vi "Set Limits on Configure Device.vi"(8 "error in (no error)":errorcluster, 10 "cluster":T1, 11 "Toggle 6 in":refnum<class "Toggle 6.lvclass">) -> (0 "error out":errorcluster, 3 "Toggle 6 out":refnum<class "Toggle 6.lvclass">)   [LabVIEW 2020, in "Toggle 6.lvclass"]
uses:
  Toggle 6.lvclass
  C:/Sandbox/Git_Sandbox/WiSpry Test Framework source code (LV20)/WiSpry Test Framework/Devices/Device.lvclass
  Controls/Configure decive refs cluster.ctl
  Controls/EFuse modes enum.ctl
  Controls/Set limt states.ctl
  <vilib>/Utility/miscctls.llb/LVMinMaxIncTypeDef.ctl
  <vilib>/Utility/miscctls.llb/LVOutOfRangeActionTypeDef.ctl
  Instruments/Power Supply/Power Supply.lvclass
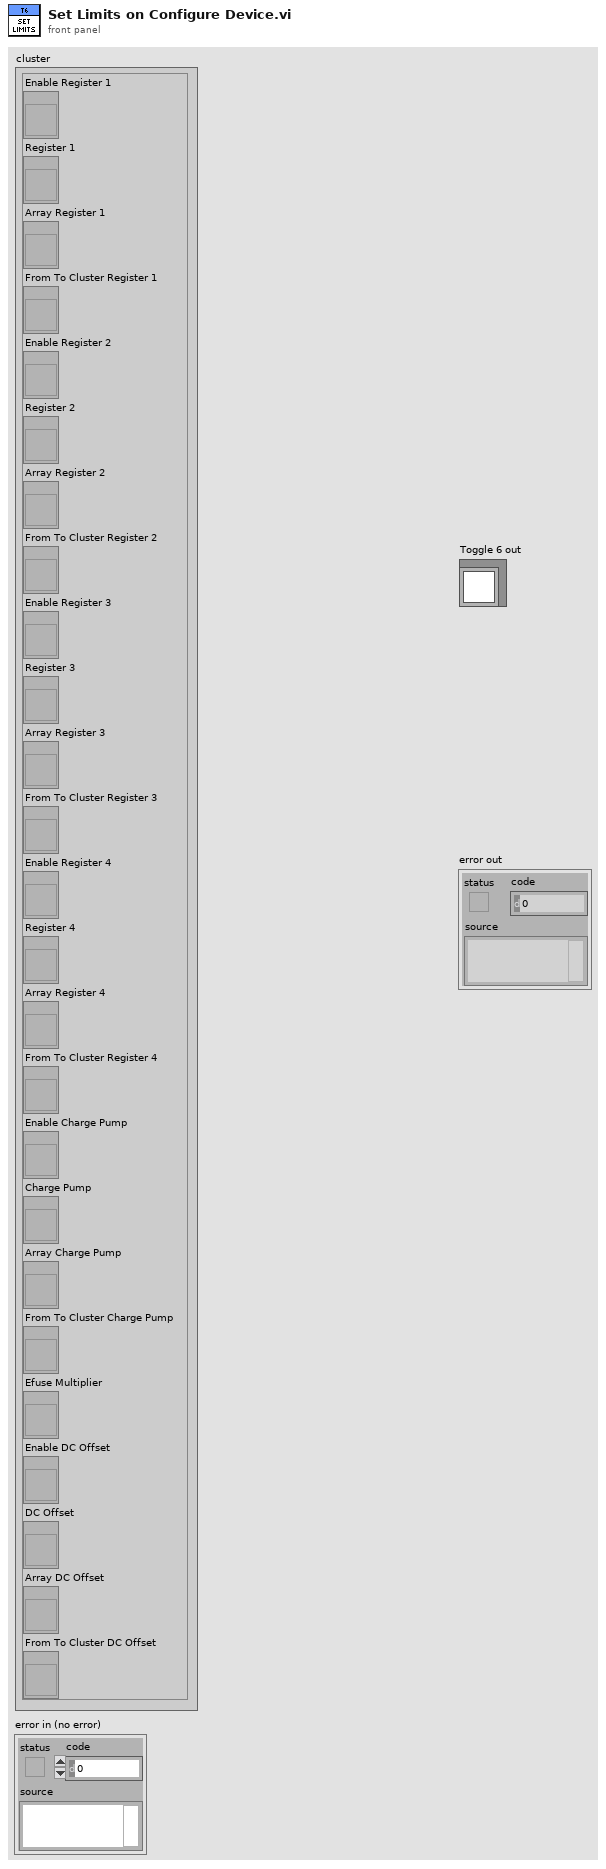
[diagram p1: front panel]
types:
  T1 = typedef "Toggle 6.lvclass/Configure decive refs cluster.ctl" = cluster{"Enable Register 1":refnum<vi>, "Register 1":refnum<vi>, "Array Register 1":refnum<vi>, "From To Cluster Register 1":refnum<vi>, "Enable Register 2":refnum<vi>, "Register 2":refnum<vi>, "Array Register 2":refnum<vi>, "From To Cluster Register 2":refnum<vi>, "Enable Register 3":refnum<vi>, "Register 3":refnum<vi>, "Array Register 3":refnum<vi>, "From To Cluster Register 3":refnum<vi>, "Enable Register 4":refnum<vi>, "Register 4":refnum<vi>, "Array Register 4":refnum<vi>, "From To Cluster Register 4":refnum<vi>, "Enable Charge Pump":refnum<vi>, "Charge Pump":refnum<vi>, "Array Charge Pump":refnum<vi>, "From To Cluster Charge Pump":refnum<vi>, "Efuse Multiplier":refnum<vi>, "Enable DC Offset":refnum<vi>, "DC Offset":refnum<vi>, "Array DC Offset":refnum<vi>, "From To Cluster DC Offset":refnum<vi>}
  T2 = typedef "Toggle 6.lvclass/Capacitor register.ctl" = cluster{"Register":u32, "Beam":dbl, "Trimmer":dbl}
  T3 = typedef "Toggle 6.lvclass/Set limt states.ctl" = enum16{"Reg 1", "Reg 2", "Reg 3", "Reg 4", "CP", "Efuse", "DC Offset", "Info", "Done"}
  T4 = typedef "LVOutOfRangeActionTypeDef.ctl" = cluster{"Out of Range Action Minimum":u8, "Out of Range Action Maximum":u8, "Out of Range Action Increment":u8}
  T5 = typedef "LVMinMaxIncTypeDef.ctl" = cluster{"Minimum":dbl, "Maximum":dbl, "Increment":dbl}
  T6 = enum8{"Enabled", "Disabled", "Disabled and Grayed Out"}
  T7 = typedef "Toggle 6.lvclass/Parameter Cluster.ctl" = cluster{"Enable":bool, "Register Number":u32, "Use Array":bool, "Array":dbl[], "To From Cluster":cluster{"From":dbl, "To":dbl, "Step":dbl}}
  T8 = typedef "Toggle 6.lvclass/Charge Pump Information cluster.ctl" = cluster{"Min":dbl, "Max":dbl, "Step":dbl, "Default":dbl}
  T9 = typedef "Toggle 6.lvclass/EFuse modes enum.ctl" = enum16{"On", "Off", "Both On and Off"}
  T10 = typedef "Device.lvclass/DC Offset Cluster.ctl" = cluster{"Enable":bool, "Use Array":bool, "Array":dbl[], "To From Cluster":cluster{"From":dbl, "To":dbl, "Step":dbl}, "Current Value":dbl, "DC Offset":refnum<class "Power Supply.lvclass">}
  T11 = typedef "Device.lvclass/Device Information Cluster.ctl" = cluster{"Device Info":string[][], "Default Values":T12[], "Fetched info":string[][]}
  T12 = typedef "PIC-Device.lvclass/Register to Write.ctl" = cluster{"Register":u32, "Value":u32, "Dev Address":u32, "Physical Adress":u32}
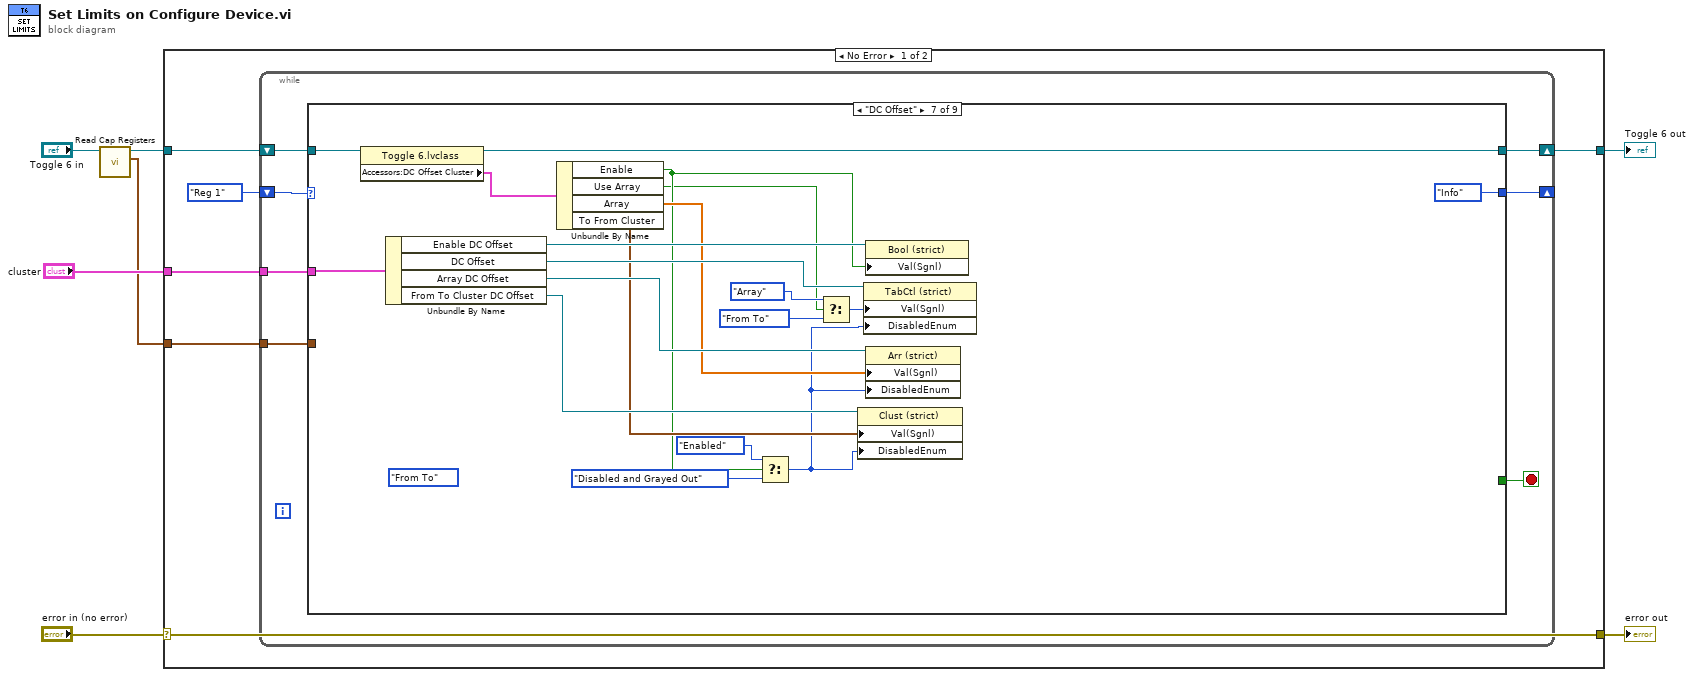
[diagram p0: block diagram]
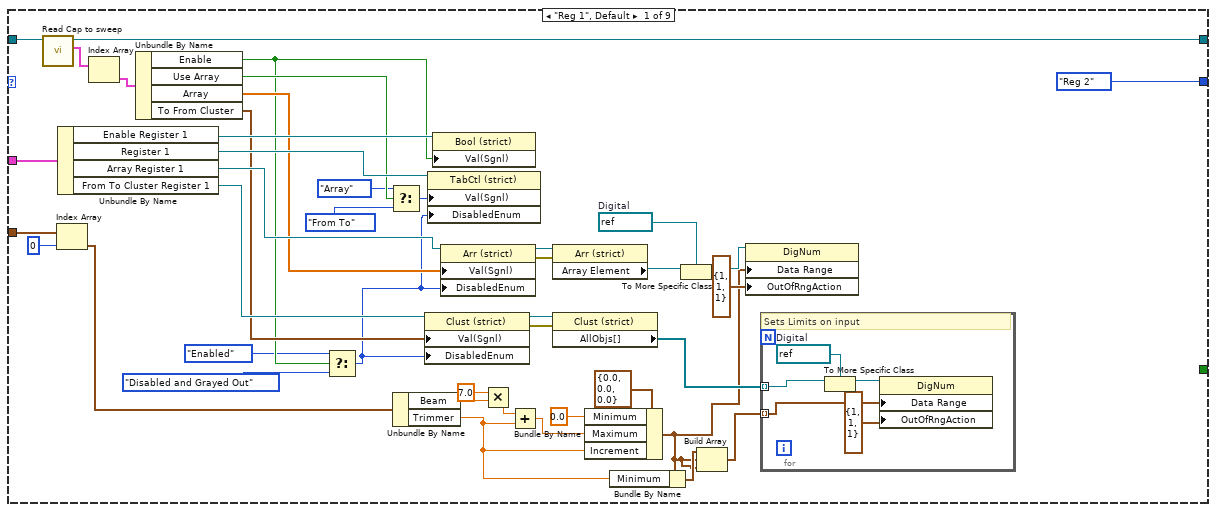
[diagram p2: hidden frame]
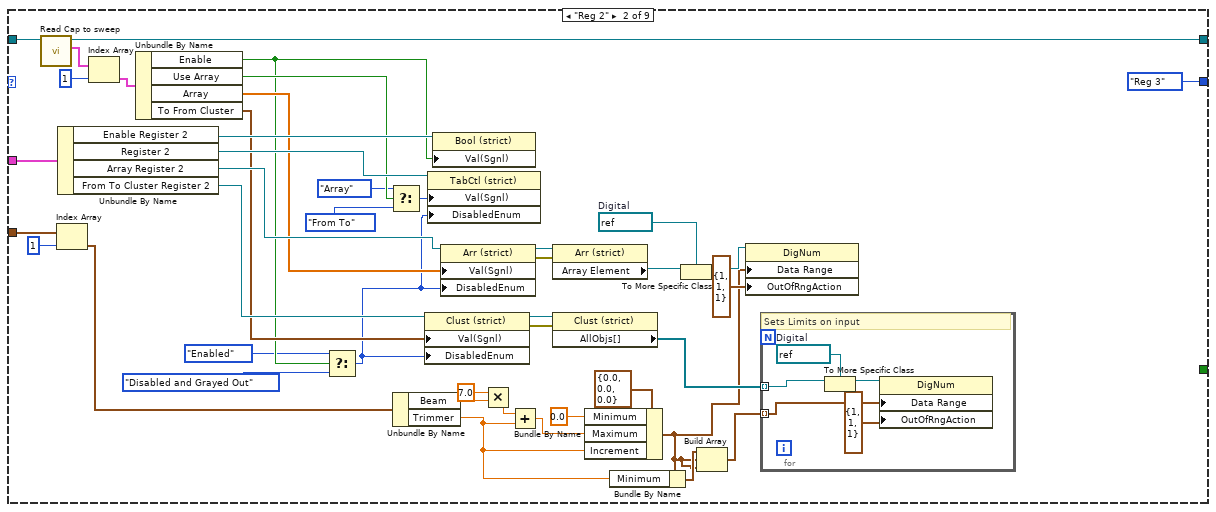
[diagram p3: hidden frame]
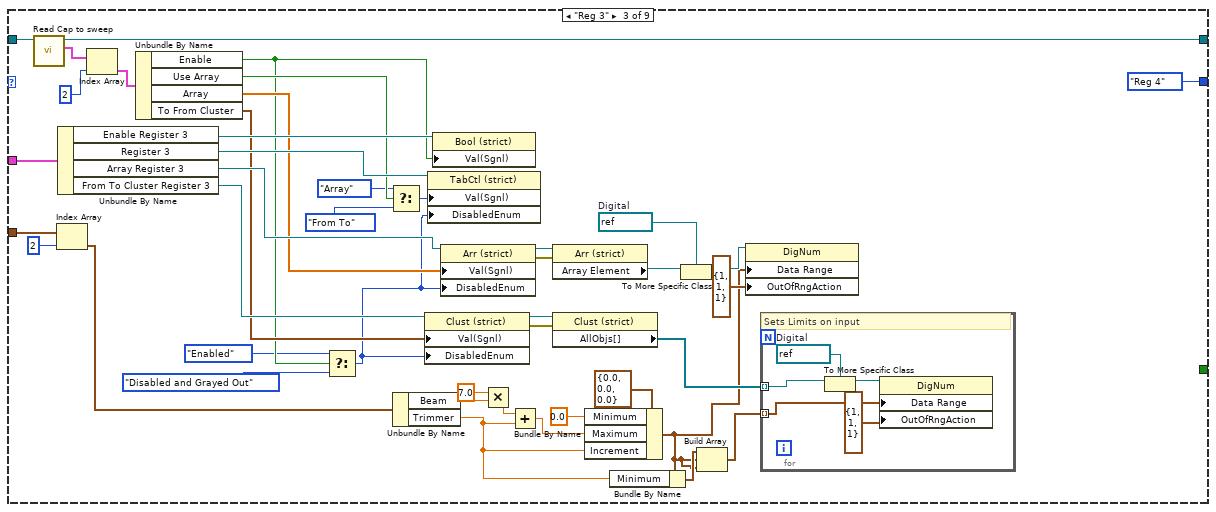
[diagram p4: hidden frame]
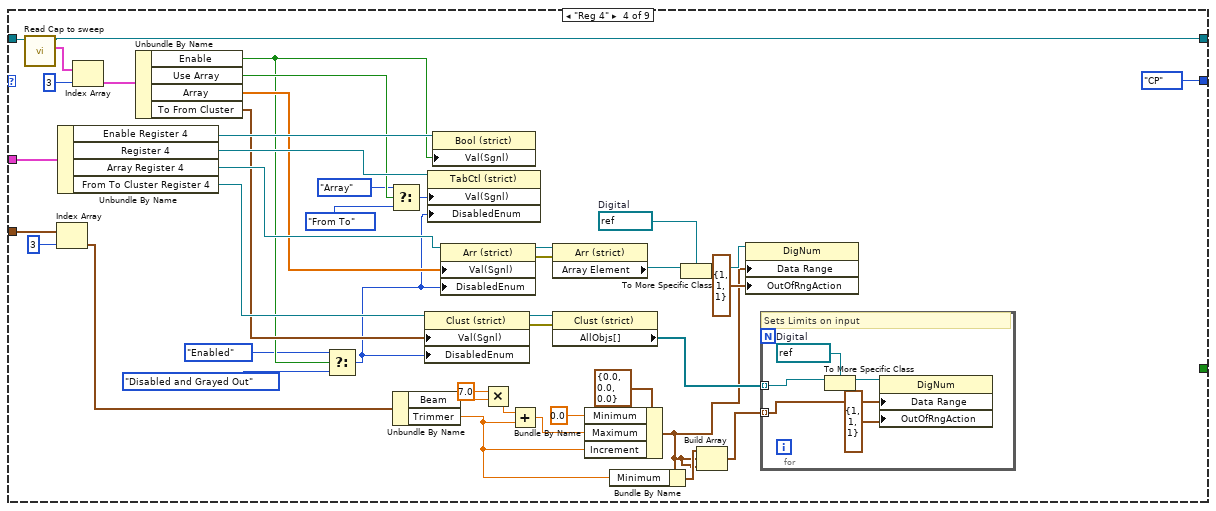
[diagram p5: hidden frame]
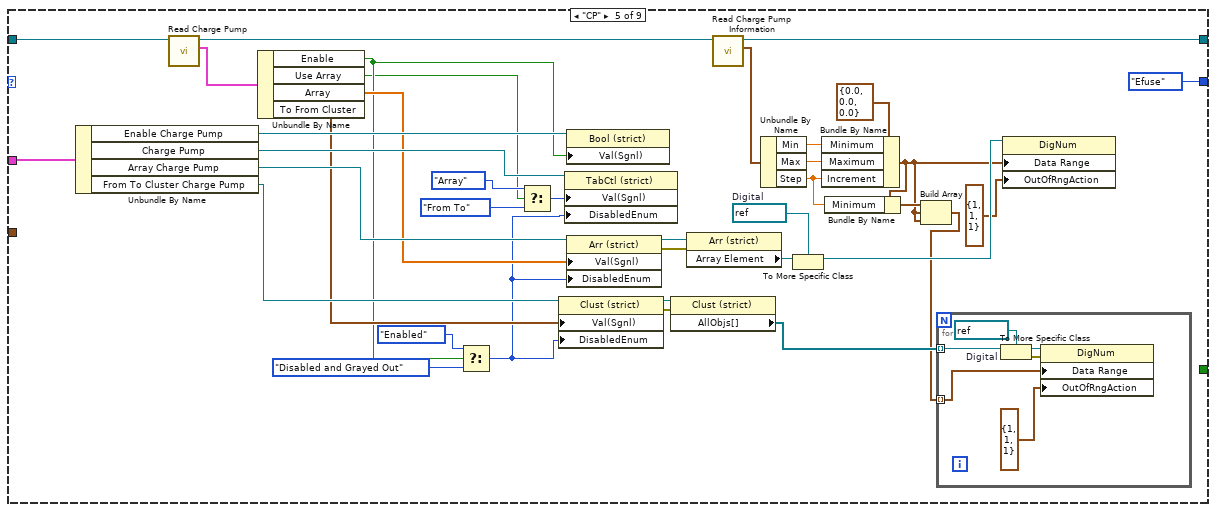
[diagram p6: hidden frame]
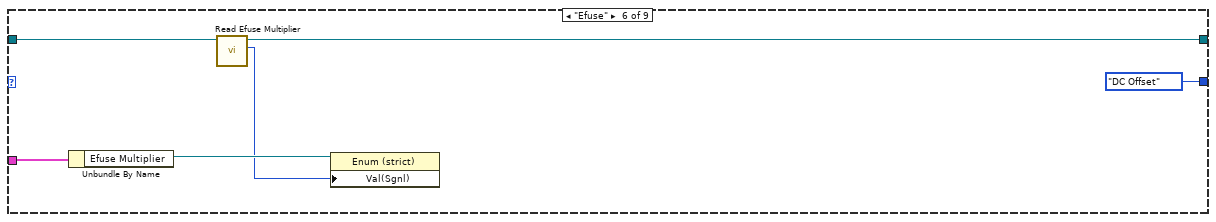
[diagram p7: hidden frame]
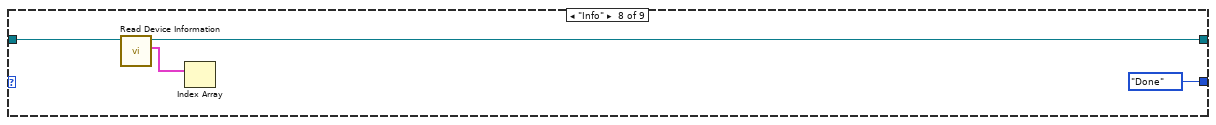
[diagram p8: hidden frame]
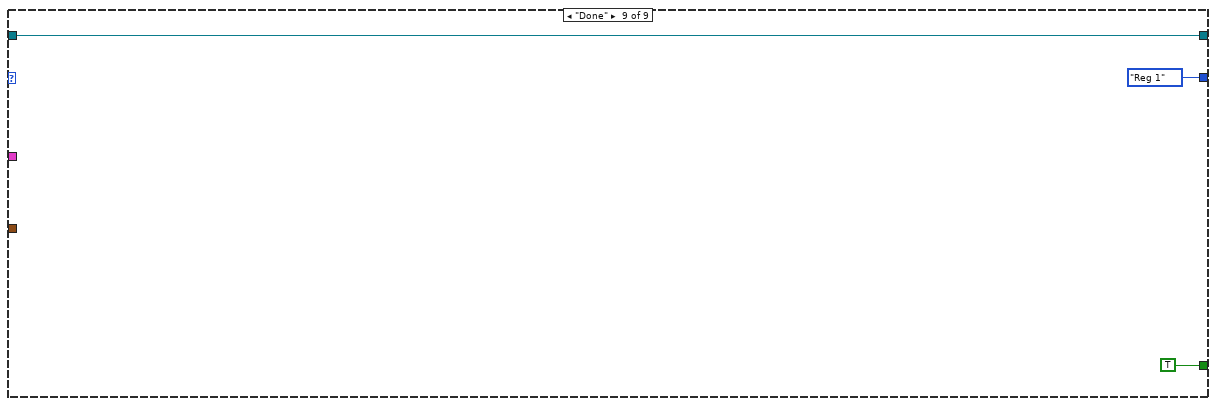
[diagram p9: hidden frame]
diagram:
  n1 = call-dynamic "Read Cap Registers.vi"("Toggle 6 in"="Toggle 6 in") -> ("Cap Registers"=w1:T2[], "Toggle 6 out"=w2:refnum<class "Toggle 6.lvclass">)  [unwired: 9 in]
  n2 = case shown="No Error" "error in (no error)" {
    selector: "error in (no error)" -> [w13 w288]
    tunnel: [w13 w288] -> w6
    tunnel: [w8 w287] -> w5
    tunnel: w2 -> [w12 w287]
    tunnel: "cluster" -> [w11 _]
    tunnel: w1 -> [w9 _]
    frame No Error {
      n3 = while {
        tunnel: w11 -> [w19]
        shift-right: [w17] -> w8
        shift-left: w12 -> [w20]
        shift-right: [w15] -> _
        shift-left: Set_limt_states."Reg 1" -> [w18]
        tunnel: w9 -> [w16]
        stop <- w14 stop-if-true
        n4 = case shown="\"DC Offset\"" w18 {
          tunnel: w20 -> [w25 w73 w121 w168 w248 w259 w263 w283 w286]
          tunnel: w19 -> [w62 w110 w158 w206 w247 w260 w279 _ _]
          tunnel: [w24 w72 w120 w169 w226 w258 w261 w281 w286] -> w17
          tunnel: w16 -> [w47 w95 w143 w191 _ _ _ _ _]
          tunnel: [Set_limt_states."Reg 2" Set_limt_states."Reg 3" Set_limt_states."Reg 4" Set_limt_states."CP" Set_limt_states."Efuse" Set_limt_states."DC Offset" Set_limt_states."Info" Set_limt_states."Done" Set_limt_states."Reg 1"] -> w15
          tunnel: [_ _ _ _ _ _ _ _ TRUE] -> w14
          frame "Reg 1", Default {
            w30 = refnum<vi> refnum  # Digital
            n5 = call-dynamic "Read Cap to sweep.vi"("Toggle 6 in"=w25) -> ("Cap to sweep"=w23:T7[], "Toggle 6 out"=w24:refnum<class "Toggle 6.lvclass">)  [unwired: 9 in]
            n6 = Index Array(array=w47, index=0) -> (element=w45:T2)
            n7 = Unbundle By Name(w62) -> ("Enable Register 1"=w61:refnum<vi>, "Register 1"=w60:refnum<vi>, "Array Register 1"=w55:refnum<vi>, "From To Cluster Register 1"=w53:refnum<vi>)
            n8 = Index Array(array=w23) -> (element=w22:T7)  [unwired: 1 in]
            n9 = Unbundle By Name(w22) -> ("Enable"=w51:bool, "Use Array"=w58:bool, "Array"=w54:dbl[], "To From Cluster"=w52:cluster{"From":dbl, "To":dbl, "Step":dbl})
            n10 = Select(t=T6."Enabled" ("Disabled"), s=w51, f=T6."Disabled and Grayed Out" ("Disabled")) -> (s? t:f=w48:T6)
            n11 = Select(t=enum32{"From To", "Array"}."Array", s=w58, f=enum32{"From To", "Array"}."From To" ("Value (Signaling)")) -> (s? t:f=w59:enum32{"From To", "Array"})
            n12 = Unbundle By Name(w45) -> ("Beam"=w41:dbl, "Trimmer"=w35:dbl)
            n13 = property class="Clust (strict)"(reference=w53, "Val(Sgnl)"=w52, "DisabledEnum"=w48) -> (reference out=w44:refnum<vi>, error out=w43:errorcluster)  [unwired: 1 in]
            n14 = property class="TabCtl (strict)"(reference=w60, "Val(Sgnl)"=w59, "DisabledEnum"=w48) -> ()  [unwired: 1 in, 2 out]
            n15 = property class="Bool (strict)"(reference=w61, "Val(Sgnl)"=w51) -> ()  [unwired: 1 in, 2 out]
            n16 = property class="Arr (strict)"(reference=w55, "Val(Sgnl)"=w54, "DisabledEnum"=w48) -> (reference out=w33:refnum<vi>, error out=w32:errorcluster)  [unwired: 1 in]
            n17 = Multiply(x=7.0, y=w41) -> (x*y=w37:dbl)
            n18 = Add(x=w37, y=w35) -> (x+y=w36:dbl)
            n19 = property class="Arr (strict)"(reference=w33, error in=w32) -> ("Array Element"=w31:refnum<vi>)  [unwired: 2 out]
            n20 = property class="Clust (strict)"(reference=w44, error in=w43) -> ("AllObjs[]"=w42:refnum<vi>[])  [unwired: 2 out]
            n21 = Bundle By Name(cluster=T5 {"Minimum"=0.0, "Maximum"=0.0, "Increment"=0.0} ("Data Entry Limits"), "Minimum"=0.0, "Maximum"=w36, "Increment"=w35) -> (w26:T5)
            n22 = Bundle By Name(cluster=w26, "Minimum"=w35) -> (w27:T5)
            n23 = To More Specific Class(target class=w30, reference=w31) -> (specific class reference=w29:refnum<vi>)  [unwired: 1 in, 1 out]
            n24 = Build Array(w27, w26, w26) -> (w34:T5[])
            n25 = property class="DigNum"(reference=w29, "Data Range"=w26, "OutOfRngAction"=T4 {"Out of Range Action Minimum"=1, "Out of Range Action Maximum"=1, "Out of Range Action Increment"=1} ("Response to Value Outside Limits")) -> ()  [unwired: 1 in, 2 out]
            n26 = for {
              tunnel: w42 -> [w66] mode=indexing
              tunnel: w34 -> [w64] mode=indexing
              w67 = refnum<vi> refnum  # Digital
              # "Sets Limits on input"
              n27 = To More Specific Class(target class=w67, reference=w66) -> (specific class reference=w65:refnum<vi>)  [unwired: 1 in, 1 out]
              n28 = property class="DigNum"(reference=w65, "Data Range"=w64, "OutOfRngAction"=T4 {"Out of Range Action Minimum"=1, "Out of Range Action Maximum"=1, "Out of Range Action Increment"=1} ("Response to Value Outside Limits")) -> ()  [unwired: 1 in, 2 out]
            }
          }
          frame "Reg 2" {
            w78 = refnum<vi> refnum  # Digital
            n29 = call-dynamic "Read Cap to sweep.vi"("Toggle 6 in"=w73) -> ("Cap to sweep"=w71:T7[], "Toggle 6 out"=w72:refnum<class "Toggle 6.lvclass">)  [unwired: 9 in]
            n30 = Index Array(array=w95, index=1) -> (element=w93:T2)
            n31 = Unbundle By Name(w110) -> ("Enable Register 2"=w109:refnum<vi>, "Register 2"=w108:refnum<vi>, "Array Register 2"=w103:refnum<vi>, "From To Cluster Register 2"=w101:refnum<vi>)
            n32 = Index Array(array=w71, index=1) -> (element=w69:T7)
            n33 = Unbundle By Name(w69) -> ("Enable"=w99:bool, "Use Array"=w106:bool, "Array"=w102:dbl[], "To From Cluster"=w100:cluster{"From":dbl, "To":dbl, "Step":dbl})
            n34 = Select(t=T6."Enabled" ("Disabled"), s=w99, f=T6."Disabled and Grayed Out" ("Disabled")) -> (s? t:f=w96:T6)
            n35 = Select(t=enum32{"From To", "Array"}."Array", s=w106, f=enum32{"From To", "Array"}."From To" ("Value (Signaling)")) -> (s? t:f=w107:enum32{"From To", "Array"})
            n36 = Unbundle By Name(w93) -> ("Beam"=w89:dbl, "Trimmer"=w83:dbl)
            n37 = property class="Clust (strict)"(reference=w101, "Val(Sgnl)"=w100, "DisabledEnum"=w96) -> (reference out=w92:refnum<vi>, error out=w91:errorcluster)  [unwired: 1 in]
            n38 = property class="TabCtl (strict)"(reference=w108, "Val(Sgnl)"=w107, "DisabledEnum"=w96) -> ()  [unwired: 1 in, 2 out]
            n39 = property class="Bool (strict)"(reference=w109, "Val(Sgnl)"=w99) -> ()  [unwired: 1 in, 2 out]
            n40 = property class="Arr (strict)"(reference=w103, "Val(Sgnl)"=w102, "DisabledEnum"=w96) -> (reference out=w81:refnum<vi>, error out=w80:errorcluster)  [unwired: 1 in]
            n41 = Multiply(x=7.0, y=w89) -> (x*y=w85:dbl)
            n42 = Add(x=w85, y=w83) -> (x+y=w84:dbl)
            n43 = property class="Arr (strict)"(reference=w81, error in=w80) -> ("Array Element"=w79:refnum<vi>)  [unwired: 2 out]
            n44 = property class="Clust (strict)"(reference=w92, error in=w91) -> ("AllObjs[]"=w90:refnum<vi>[])  [unwired: 2 out]
            n45 = Bundle By Name(cluster=T5 {"Minimum"=0.0, "Maximum"=0.0, "Increment"=0.0} ("Data Entry Limits"), "Minimum"=0.0, "Maximum"=w84, "Increment"=w83) -> (w74:T5)
            n46 = Bundle By Name(cluster=w74, "Minimum"=w83) -> (w75:T5)
            n47 = To More Specific Class(target class=w78, reference=w79) -> (specific class reference=w77:refnum<vi>)  [unwired: 1 in, 1 out]
            n48 = Build Array(w75, w74, w74) -> (w82:T5[])
            n49 = property class="DigNum"(reference=w77, "Data Range"=w74, "OutOfRngAction"=T4 {"Out of Range Action Minimum"=1, "Out of Range Action Maximum"=1, "Out of Range Action Increment"=1} ("Response to Value Outside Limits")) -> ()  [unwired: 1 in, 2 out]
            n50 = for {
              tunnel: w90 -> [w114] mode=indexing
              tunnel: w82 -> [w112] mode=indexing
              w115 = refnum<vi> refnum  # Digital
              # "Sets Limits on input"
              n51 = To More Specific Class(target class=w115, reference=w114) -> (specific class reference=w113:refnum<vi>)  [unwired: 1 in, 1 out]
              n52 = property class="DigNum"(reference=w113, "Data Range"=w112, "OutOfRngAction"=T4 {"Out of Range Action Minimum"=1, "Out of Range Action Maximum"=1, "Out of Range Action Increment"=1} ("Response to Value Outside Limits")) -> ()  [unwired: 1 in, 2 out]
            }
          }
          frame "Reg 3" {
            w126 = refnum<vi> refnum  # Digital
            n53 = call-dynamic "Read Cap to sweep.vi"("Toggle 6 in"=w121) -> ("Cap to sweep"=w119:T7[], "Toggle 6 out"=w120:refnum<class "Toggle 6.lvclass">)  [unwired: 9 in]
            n54 = Index Array(array=w143, index=2) -> (element=w141:T2)
            n55 = Unbundle By Name(w158) -> ("Enable Register 3"=w157:refnum<vi>, "Register 3"=w156:refnum<vi>, "Array Register 3"=w151:refnum<vi>, "From To Cluster Register 3"=w149:refnum<vi>)
            n56 = Index Array(array=w119, index=2) -> (element=w118:T7)
            n57 = Unbundle By Name(w118) -> ("Enable"=w147:bool, "Use Array"=w154:bool, "Array"=w150:dbl[], "To From Cluster"=w148:cluster{"From":dbl, "To":dbl, "Step":dbl})
            n58 = Select(t=T6."Enabled" ("Disabled"), s=w147, f=T6."Disabled and Grayed Out" ("Disabled")) -> (s? t:f=w144:T6)
            n59 = Select(t=enum32{"From To", "Array"}."Array", s=w154, f=enum32{"From To", "Array"}."From To" ("Value (Signaling)")) -> (s? t:f=w155:enum32{"From To", "Array"})
            n60 = Unbundle By Name(w141) -> ("Beam"=w137:dbl, "Trimmer"=w131:dbl)
            n61 = property class="Clust (strict)"(reference=w149, "Val(Sgnl)"=w148, "DisabledEnum"=w144) -> (reference out=w140:refnum<vi>, error out=w139:errorcluster)  [unwired: 1 in]
            n62 = property class="TabCtl (strict)"(reference=w156, "Val(Sgnl)"=w155, "DisabledEnum"=w144) -> ()  [unwired: 1 in, 2 out]
            n63 = property class="Bool (strict)"(reference=w157, "Val(Sgnl)"=w147) -> ()  [unwired: 1 in, 2 out]
            n64 = property class="Arr (strict)"(reference=w151, "Val(Sgnl)"=w150, "DisabledEnum"=w144) -> (reference out=w129:refnum<vi>, error out=w128:errorcluster)  [unwired: 1 in]
            n65 = Multiply(x=7.0, y=w137) -> (x*y=w133:dbl)
            n66 = Add(x=w133, y=w131) -> (x+y=w132:dbl)
            n67 = property class="Arr (strict)"(reference=w129, error in=w128) -> ("Array Element"=w127:refnum<vi>)  [unwired: 2 out]
            n68 = property class="Clust (strict)"(reference=w140, error in=w139) -> ("AllObjs[]"=w138:refnum<vi>[])  [unwired: 2 out]
            n69 = Bundle By Name(cluster=T5 {"Minimum"=0.0, "Maximum"=0.0, "Increment"=0.0} ("Data Entry Limits"), "Minimum"=0.0, "Maximum"=w132, "Increment"=w131) -> (w122:T5)
            n70 = Bundle By Name(cluster=w122, "Minimum"=w131) -> (w123:T5)
            n71 = To More Specific Class(target class=w126, reference=w127) -> (specific class reference=w125:refnum<vi>)  [unwired: 1 in, 1 out]
            n72 = Build Array(w123, w122, w122) -> (w130:T5[])
            n73 = property class="DigNum"(reference=w125, "Data Range"=w122, "OutOfRngAction"=T4 {"Out of Range Action Minimum"=1, "Out of Range Action Maximum"=1, "Out of Range Action Increment"=1} ("Response to Value Outside Limits")) -> ()  [unwired: 1 in, 2 out]
            n74 = for {
              tunnel: w138 -> [w162] mode=indexing
              tunnel: w130 -> [w160] mode=indexing
              w163 = refnum<vi> refnum  # Digital
              # "Sets Limits on input"
              n75 = To More Specific Class(target class=w163, reference=w162) -> (specific class reference=w161:refnum<vi>)  [unwired: 1 in, 1 out]
              n76 = property class="DigNum"(reference=w161, "Data Range"=w160, "OutOfRngAction"=T4 {"Out of Range Action Minimum"=1, "Out of Range Action Maximum"=1, "Out of Range Action Increment"=1} ("Response to Value Outside Limits")) -> ()  [unwired: 1 in, 2 out]
            }
          }
          frame "Reg 4" {
            w174 = refnum<vi> refnum  # Digital
            n77 = call-dynamic "Read Cap to sweep.vi"("Toggle 6 in"=w168) -> ("Cap to sweep"=w167:T7[], "Toggle 6 out"=w169:refnum<class "Toggle 6.lvclass">)  [unwired: 9 in]
            n78 = Index Array(array=w191, index=3) -> (element=w189:T2)
            n79 = Unbundle By Name(w206) -> ("Enable Register 4"=w205:refnum<vi>, "Register 4"=w204:refnum<vi>, "Array Register 4"=w199:refnum<vi>, "From To Cluster Register 4"=w197:refnum<vi>)
            n80 = Index Array(array=w167, index=3) -> (element=w166:T7)
            n81 = Unbundle By Name(w166) -> ("Enable"=w195:bool, "Use Array"=w202:bool, "Array"=w198:dbl[], "To From Cluster"=w196:cluster{"From":dbl, "To":dbl, "Step":dbl})
            n82 = Select(t=T6."Enabled" ("Disabled"), s=w195, f=T6."Disabled and Grayed Out" ("Disabled")) -> (s? t:f=w192:T6)
            n83 = Select(t=enum32{"From To", "Array"}."Array", s=w202, f=enum32{"From To", "Array"}."From To" ("Value (Signaling)")) -> (s? t:f=w203:enum32{"From To", "Array"})
            n84 = Unbundle By Name(w189) -> ("Beam"=w185:dbl, "Trimmer"=w179:dbl)
            n85 = property class="Clust (strict)"(reference=w197, "Val(Sgnl)"=w196, "DisabledEnum"=w192) -> (reference out=w188:refnum<vi>, error out=w187:errorcluster)  [unwired: 1 in]
            n86 = property class="TabCtl (strict)"(reference=w204, "Val(Sgnl)"=w203, "DisabledEnum"=w192) -> ()  [unwired: 1 in, 2 out]
            n87 = property class="Bool (strict)"(reference=w205, "Val(Sgnl)"=w195) -> ()  [unwired: 1 in, 2 out]
            n88 = property class="Arr (strict)"(reference=w199, "Val(Sgnl)"=w198, "DisabledEnum"=w192) -> (reference out=w177:refnum<vi>, error out=w176:errorcluster)  [unwired: 1 in]
            n89 = Multiply(x=7.0, y=w185) -> (x*y=w181:dbl)
            n90 = Add(x=w181, y=w179) -> (x+y=w180:dbl)
            n91 = property class="Arr (strict)"(reference=w177, error in=w176) -> ("Array Element"=w175:refnum<vi>)  [unwired: 2 out]
            n92 = property class="Clust (strict)"(reference=w188, error in=w187) -> ("AllObjs[]"=w186:refnum<vi>[])  [unwired: 2 out]
            n93 = Bundle By Name(cluster=T5 {"Minimum"=0.0, "Maximum"=0.0, "Increment"=0.0} ("Data Entry Limits"), "Minimum"=0.0, "Maximum"=w180, "Increment"=w179) -> (w170:T5)
            n94 = Bundle By Name(cluster=w170, "Minimum"=w179) -> (w171:T5)
            n95 = To More Specific Class(target class=w174, reference=w175) -> (specific class reference=w173:refnum<vi>)  [unwired: 1 in, 1 out]
            n96 = Build Array(w171, w170, w170) -> (w178:T5[])
            n97 = property class="DigNum"(reference=w173, "Data Range"=w170, "OutOfRngAction"=T4 {"Out of Range Action Minimum"=1, "Out of Range Action Maximum"=1, "Out of Range Action Increment"=1} ("Response to Value Outside Limits")) -> ()  [unwired: 1 in, 2 out]
            n98 = for {
              tunnel: w186 -> [w210] mode=indexing
              tunnel: w178 -> [w208] mode=indexing
              w211 = refnum<vi> refnum  # Digital
              # "Sets Limits on input"
              n99 = To More Specific Class(target class=w211, reference=w210) -> (specific class reference=w209:refnum<vi>)  [unwired: 1 in, 1 out]
              n100 = property class="DigNum"(reference=w209, "Data Range"=w208, "OutOfRngAction"=T4 {"Out of Range Action Minimum"=1, "Out of Range Action Maximum"=1, "Out of Range Action Increment"=1} ("Response to Value Outside Limits")) -> ()  [unwired: 1 in, 2 out]
            }
          }
          frame "CP" {
            w229 = refnum<vi> refnum  # Digital
            n101 = Unbundle By Name(w247) -> ("Enable Charge Pump"=w245:refnum<vi>, "Charge Pump"=w244:refnum<vi>, "Array Charge Pump"=w240:refnum<vi>, "From To Cluster Charge Pump"=w238:refnum<vi>)
            n102 = call-dynamic "Read Charge Pump.vi"("Toggle 6 in"=w248) -> ("Parameter Cluster"=w246:T7, "Toggle 6 out"=w227:refnum<class "Toggle 6.lvclass">)  [unwired: 8 in, 1 out]
            n103 = Unbundle By Name(w246) -> ("Enable"=w236:bool, "Use Array"=w212:bool, "Array"=w239:dbl[], "To From Cluster"=w237:cluster{"From":dbl, "To":dbl, "Step":dbl})
            n104 = Select(t=T6."Enabled" ("Disabled"), s=w236, f=T6."Disabled and Grayed Out") -> (s? t:f=w233:T6)
            n105 = Select(t=enum32{"From To", "Array"}."Array" ("Value (Signaling)"), s=w212, f=enum32{"From To", "Array"}."From To") -> (s? t:f=w242:enum32{"From To", "Array"})
            n106 = property class="Clust (strict)"(reference=w238, "Val(Sgnl)"=w237, "DisabledEnum"=w233) -> (reference out=w221:refnum<vi>, error out=w220:errorcluster)  [unwired: 1 in]
            n107 = property class="TabCtl (strict)"(reference=w244, "Val(Sgnl)"=w242, "DisabledEnum"=w233) -> ()  [unwired: 1 in, 2 out]
            n108 = property class="Bool (strict)"(reference=w245, "Val(Sgnl)"=w236) -> ()  [unwired: 1 in, 2 out]
            n109 = property class="Arr (strict)"(reference=w240, "Val(Sgnl)"=w239, "DisabledEnum"=w233) -> (reference out=w232:refnum<vi>, error out=w231:errorcluster)  [unwired: 1 in]
            n110 = property class="Clust (strict)"(reference=w221, error in=w220) -> ("AllObjs[]"=w219:refnum<vi>[])  [unwired: 2 out]
            n111 = property class="Arr (strict)"(reference=w232, error in=w231) -> ("Array Element"=w230:refnum<vi>)  [unwired: 2 out]
            n112 = call-dynamic "Read Charge Pump Information.vi"("Toggle 6 in"=w227) -> ("Charge Pump Information"=w224:T8, "Toggle 6 out"=w226:refnum<class "Toggle 6.lvclass">)  [unwired: 9 in]
            n113 = Unbundle By Name(w224) -> ("Min"=w223:dbl, "Max"=w222:dbl, "Step"=w218:dbl)
            n114 = To More Specific Class(target class=w229, reference=w230) -> (specific class reference=w228:refnum<vi>)  [unwired: 1 in, 1 out]
            n115 = Bundle By Name(cluster=T5 {"Minimum"=0.0, "Maximum"=0.0, "Increment"=0.0} ("Data Entry Limits"), "Minimum"=w223, "Maximum"=w222, "Increment"=w218) -> (w216:T5)
            n116 = Bundle By Name(cluster=w216, "Minimum"=w218) -> (w217:T5)
            n117 = Build Array(w217, w216, w216) -> (w215:T5[])
            n118 = for {
              tunnel: w219 -> [w254] mode=indexing
              tunnel: w215 -> [w250] mode=indexing
              w253 = refnum<vi> refnum  # Digital
              n119 = To More Specific Class(target class=w253, reference=w254) -> (specific class reference=w252:refnum<vi>, error out=w251:errorcluster)  [unwired: 1 in]
              n120 = property class="DigNum"(reference=w252, error in=w251, "Data Range"=w250, "OutOfRngAction"=T4 {"Out of Range Action Minimum"=1, "Out of Range Action Maximum"=1, "Out of Range Action Increment"=1} ("Response to Value Outside Limits")) -> ()  [unwired: 2 out]
            }
            n121 = property class="DigNum"(reference=w228, "Data Range"=w216, "OutOfRngAction"=T4 {"Out of Range Action Minimum"=1, "Out of Range Action Maximum"=1, "Out of Range Action Increment"=1} ("Response to Value Outside Limits")) -> ()  [unwired: 1 in, 2 out]
          }
          frame "Efuse" {
            n122 = Unbundle By Name(w260) -> ("Efuse Multiplier"=w257:refnum<vi>)
            n123 = call-dynamic "Read Efuse Multiplier.vi"("Toggle 6 in"=w259) -> ("Efuse Multiplier"=w256:T9, "Toggle 6 out"=w258:refnum<class "Toggle 6.lvclass">)  [unwired: 9 in]
            n124 = property class="Enum (strict)"(reference=w257, "Val(Sgnl)"=w256) -> ()  [unwired: 1 in, 2 out]
          }
          frame "DC Offset" {
            (unwired) enum32{"From To", "Array"}."From To" ("s? t:f")
            n125 = property class="Toggle 6.lvclass"(reference=w263) -> (reference out=w261:refnum<class "Toggle 6.lvclass">, "Accessors:DC Offset Cluster"=w262:T10)  [unwired: 1 in, 1 out]
            n126 = Unbundle By Name(w279) -> ("Enable DC Offset"=w278:refnum<vi>, "DC Offset"=w277:refnum<vi>, "Array DC Offset"=w273:refnum<vi>, "From To Cluster DC Offset"=w271:refnum<vi>)
            n127 = Unbundle By Name(w262) -> ("Enable"=w269:bool, "Use Array"=w264:bool, "Array"=w272:dbl[], "To From Cluster"=w270:cluster{"From":dbl, "To":dbl, "Step":dbl})
            n128 = Select(t=T6."Enabled" ("Disabled"), s=w269, f=T6."Disabled and Grayed Out") -> (s? t:f=w266:T6)
            n129 = Select(t=enum32{"From To", "Array"}."Array" ("Value (Signaling)"), s=w264, f=enum32{"From To", "Array"}."From To") -> (s? t:f=w275:enum32{"From To", "Array"})
            n130 = property class="Clust (strict)"(reference=w271, "Val(Sgnl)"=w270, "DisabledEnum"=w266) -> ()  [unwired: 1 in, 2 out]
            n131 = property class="TabCtl (strict)"(reference=w277, "Val(Sgnl)"=w275, "DisabledEnum"=w266) -> ()  [unwired: 1 in, 2 out]
            n132 = property class="Bool (strict)"(reference=w278, "Val(Sgnl)"=w269) -> ()  [unwired: 1 in, 2 out]
            n133 = property class="Arr (strict)"(reference=w273, "Val(Sgnl)"=w272, "DisabledEnum"=w266) -> ()  [unwired: 1 in, 2 out]
          }
          frame "Info" {
            n134 = call-dynamic "Read Device Information.vi"("Device in"=w283) -> ("Device Info"=w282:T11[], "Device out"=w281:refnum<class "Toggle 6.lvclass">)  [unwired: 8 in, 1 out]
            n135 = Index Array(array=w282) -> ()  [unwired: 1 in, 1 out]
          }
          frame "Done" {
          }
        }
      }
    }
    frame Error {
    }
  }
  "error out" <- w6
  "Toggle 6 out" <- w5
